vi "Send Launch Actors.vi"(7 "Message Priority (Normal)":T1=enum."Normal", 8 "error in (no error)":errorcluster, 10 "Selected Actors":string[](array[string]), 11 "Message Enqueuer":refnum<class "Message Enqueuer.lvclass">) -> (0 "error out":errorcluster, 3 "Message Enqueuer out":refnum<class "Message Enqueuer.lvclass">)   [LabVIEW 2015, in "CS++StartActor.lvlib" / "Launch Actors Msg.lvclass"]
doc: "Sends the <B>CS++StartActor.lvlib:Launch Actors Msg.lvclass</B> message.\n\n<B>CS++StartActor.lvlib:CS++StartActor.lvclass:Launch Actors.vi</B> Description:\n\nLaunch Start Actors."
uses:
  Launch Actors Msg.lvclass
  <vilib>/ActorFramework/Message Enqueuer/Message Enqueuer.lvclass
  <vilib>/ActorFramework/Message Enqueuer/Message Priority.ctl
  Launch Actors Msg.lvclass/Launch Actors Msg.ctl
  <vilib>/ActorFramework/Message Enqueuer/Message Enqueuer.lvclass/Message Enqueuer.ctl
  <vilib>/ActorFramework/Message Priority Queue/Priority Enqueue.vi
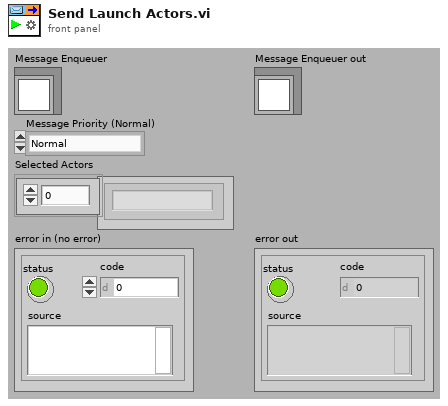
[diagram p1: front panel]
types:
  T1 = typedef "Actor Framework.lvlib/Message Enqueuer.lvclass/Message Priority.ctl" = enum16{"Low", "Normal", "High"}
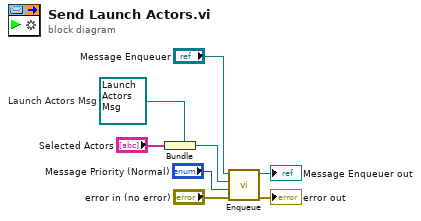
[diagram p0: block diagram]
diagram:
  w2 = refnum<class "Launch Actors Msg.lvclass"> refnum  # Launch Actors Msg
  n1 = Bundle(cluster=w2, "Selected Actors") -> (w5:refnum<class "Launch Actors Msg.lvclass">)
  n2 = call <vilib>:"Enqueue.vi"("error in (no error)"="error in (no error)", "Message Priority (Normal)"="Message Priority (Normal)", "Message"=w5, "Message Enqueuer in"="Message Enqueuer") -> ("error out"=→"error out":errorcluster, "Message Enqueuer out"=→"Message Enqueuer out":refnum<class "Message Enqueuer.lvclass">)  [unwired: 6 in]
